vi "stopTask.vi"() -> ()   [LabVIEW 2010, in "pdbm_task_route.lvlib"]
uses:
  pdbm_task_route.lvlib
panel:
  in  "error in (no error)":errorcluster
  in  "Task Ref":refnum<vi>
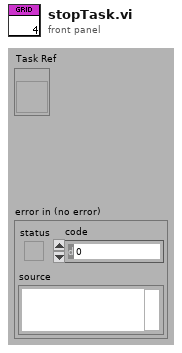
[diagram p1: front panel]
types:
  T1 = enum32{"Bad", "Idle", "Run top level", "Running"}
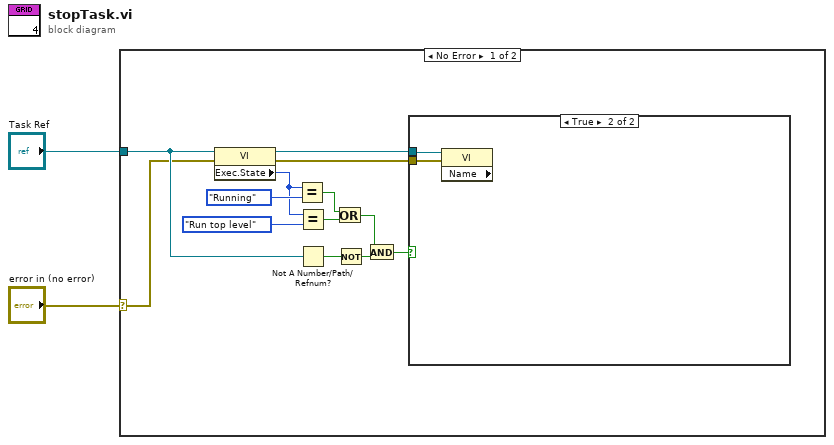
[diagram p0: block diagram]
diagram:
  n1 = case shown="No Error" "error in (no error)" {
    selector: "error in (no error)" -> [w13 _]
    tunnel: "Task Ref" -> [w14 _]
    frame No Error {
      n2 = property class="VI"(reference=w14, error in=w13) -> (reference out=w5:refnum<vi>, error out=w3:errorcluster, "Exec.State"=w11:T1)
      n3 = Equal?(x=w11, y=T1."Running") -> (x = y?=w8:bool)
      n4 = Equal?(x=w11, y=T1."Run top level") -> (x = y?=w9:bool)
      n5 = Not A Number/Path/Refnum?(number/path/refnum=w14) -> (NaN/Path/Refnum?=w15:bool)
      n6 = Or(x=w8, y=w9) -> (x .or. y?=w6:bool)
      n7 = Not(x=w15) -> (.not. x?=w7:bool)
      n8 = And(x=w6, y=w7) -> (x .and. y?=w4:bool)
      n9 = case shown="True" w4 {
        tunnel: w5 -> [_ w17]
        tunnel: w3 -> [_ w16]
        frame False {
        }
        frame True {
          n10 = property class="VI" props=["Name"](reference=w17, error in=w16) -> ()  [unwired: 3 out]
        }
      }
    }
    frame Error {
    }
  }
